vi "Send Manual Trigger.vi"(8 "error in (no error)":errorcluster, 11 "VISA resource name":refnum<visa-resource-name>) -> (0 "error out":errorcluster, 3 "VISA resource name out":refnum<visa-resource-name>)   [LabVIEW 2019, in "Agilent E4980.lvlib"]
doc: "Triggers the LCR meter, then the instrument invalidates all measurement results and starts a new measuring cycle with the current settings.\n\n<B>Notes:</B>\n(1) You have to set the trigger source as Manual, External or Bus when sending the trigger. (NOT Internal)\n\n(2) The instrument can be in \"Wait for Trigger\" or \"Idle\" state when sending the trigger."
uses:
  Agilent E4980.lvlib
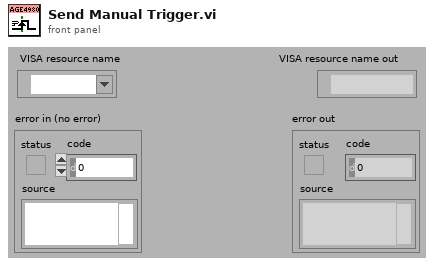
[diagram p1: front panel]
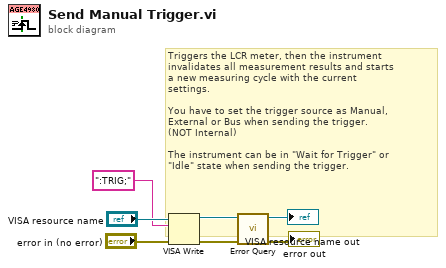
[diagram p0: block diagram]
diagram:
  # "Triggers the LCR meter, then the instrument\ninvalidates all measurement results and starts\na new measuring cycle with the current\nsettings.\n\nYou have to set the trigger source as Manual,\nExternal or Bus when sending the trigger. \n(NOT Internal)\n\nThe instrument can be in \"Wait for Trigger\" or\n\"Idle\" state when sending the trigger."
  n1 = VISA Write(VISA resource name="VISA resource name", write buffer=":TRIG;", error in (no error)="error in (no error)") -> (VISA resource name out=w2:refnum<visa-resource-name>, error out=w1:errorcluster)  [unwired: 1 out]
  n2 = call "Error Query.vi"("error in (no error)"=w1, "VISA resource name"=w2) -> ("error out"=→"error out":errorcluster, "VISA resource name out"=→"VISA resource name out":refnum<visa-resource-name>)  [unwired: 6 in, 2 out]
